vi "State_Waiting.vi"(8 "error in (no error)":errorcluster, 9 "Parameter":variant, 10 "Command":string, 11 "MB Slave Simulator Base in":refnum<class "MB Slave Simulator Base.lvclass">) -> (0 "error out":errorcluster, 2 "Debug Message":string, 3 "MB Slave Simulator Base out":refnum<class "MB Slave Simulator Base.lvclass">)   [LabVIEW 2021, in "MB Slave Simulator Base.lvclass"]
uses:
  MB Slave Simulator Base.lvclass
  C:/Program Files (x86)/National Instruments/LabVIEW 2021/user.lib/S2 Labs/Module Framework/Modules/Base/Module.lvclass
  C:/Program Files (x86)/National Instruments/LabVIEW 2021/user.lib/S2 Labs/Module Framework/Modules/Modbus/Modbus Slave Base/Modbus Slave Base.lvclass
  <userlib>/S2 Labs/CVT Toolkit/CVT.lvclass/CVT.ctl
  <userlib>/S2 Labs/Module Framework/Modules/Modbus/Modbus Slave Base/Modbus Slave Base.lvclass/Modbus Slave Base.ctl
  <userlib>/S2 Labs/Module Framework/Modules/Base/Module.lvclass/Module.ctl
  b9a700bc-881b-4d61-b18c-b62fca83ff33.vi
  d79701ff-d040-49f0-829a-e0d127d096ef.vi
  010a9ca9-5f64-4ce6-a378-2df25787252c.vi
  <userlib>/S2 Labs/Module Framework/Modules/Modbus/Modbus Slave Base/Read MB Ref.vi
  b9a700bc-881b-4d61-b18c-b62fca83ff33.vi/1553f4ce-967c-4f57-a913-5f155bf4374d.vi
  d79701ff-d040-49f0-829a-e0d127d096ef.vi/71b19a30-41bb-452f-8775-2cd3e07414b9.vi
  <userlib>/S2 Labs/Module Framework/Modules/Base/Read Module CVT.vi
  010a9ca9-5f64-4ce6-a378-2df25787252c.vi/71b19a30-41bb-452f-8775-2cd3e07414b9.vi
  <userlib>/S2 Labs/CVT Toolkit/Read CVT DVR.vi
  <userlib>/S2 Labs/CVT Toolkit/Variant Functions/Write Reserved Attributes.vi
  <userlib>/S2 Labs/CVT Toolkit/Variant Functions/Write Alias Attribute.vi
  <userlib>/S2 Labs/CVT Toolkit/Variant Functions/Write Unit Attribute.vi
  <userlib>/S2 Labs/CVT Toolkit/Variant Functions/Write Type Attribute.vi
  <userlib>/S2 Labs/CVT Toolkit/Variant Functions/Write Parms Attribute.vi
  <userlib>/S2 Labs/Module Framework/Modules/Base/Get Module CVT Ref.vi
  <userlib>/S2 Labs/Module Framework/Modules/Base/Trigger Logging Write.vi
  <userlib>/S2 Labs/Modbus Toolkit/Slave/S2L Modbus Slave.lvclass
  <userlib>/S2 Labs/CVT Toolkit/CVT.lvclass
  MB Slave Simulator Base.lvclass/MB Slave Simulator Base.ctl
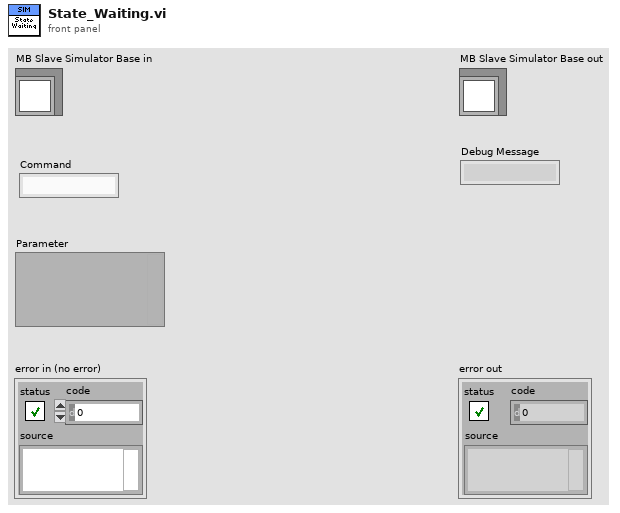
[diagram p1: front panel]
types:
  T1 = cluster{"daemon status":enum16{"Not Started", "Running", "Error", "Stopped"}, "daemon error":errorcluster, "connection count":u32, "connections":cluster{"Connected?":bool, "IP address":string, "connection error":errorcluster}[]}
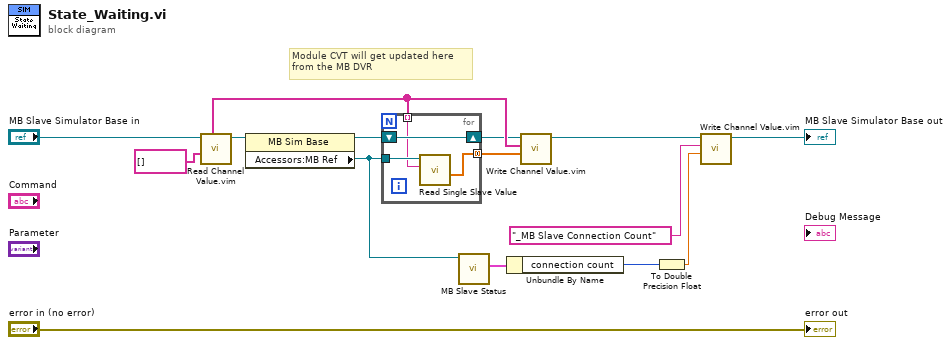
[diagram p0: block diagram]
diagram:
  # "Module CVT will get updated here\nfrom the MB DVR"
  n1 = call "Read Channel Value.vim"("Channel Label(s)"=string[] [], "Module in"="MB Slave Simulator Base in") -> ("Module out"=w9:refnum<class "MB Slave Simulator Base.lvclass">, "Channel Labels*"=w12:string[])  [unwired: 3 in, 5 out]
  n2 = property class="MB Sim Base"(reference=w9) -> (reference out=w10:refnum<class "MB Slave Simulator Base.lvclass">, "Accessors:MB Ref"=w15:refnum<class "S2L Modbus Slave.lvclass">)  [unwired: 1 in, 1 out]
  n3 = for {
    tunnel: w15 -> [w19]
    shift-right: [w18] -> w11
    shift-left: w10 -> [w18]
    tunnel: w12 -> [w17] mode=indexing
    tunnel: [w16] -> w13 mode=concatenating
    n4 = call-dynamic "Read Single Slave Value.vi"("Label"=w17, "S2L Modbus Slave in"=w19) -> ("Value (s)"=w16:dbl[])  [unwired: 4 in, 5 out]
  }
  n5 = call <userlib>:"MB Slave Status.vi"("S2L Modbus Slave in"=w15) -> ("MB Slave Status"=w4:T1)  [unwired: 8 in, 2 out]
  n6 = Unbundle By Name(w4) -> ("connection count"=w6:u32)
  n7 = call "Write Channel Value.vim"("value"=w13, "Channel Label(s)"=w12, "Module in"=w11) -> ("Module out"=w14:refnum<class "MB Slave Simulator Base.lvclass">)  [unwired: 6 in, 2 out]
  n8 = To Double Precision Float(number=w6) -> (double precision float=w7:dbl)
  n9 = call "Write Channel Value.vim"("value"=w7, "Channel Label(s)"="_MB Slave Connection Count", "Module in"=w14) -> ("Module out"=→"MB Slave Simulator Base out":refnum<class "MB Slave Simulator Base.lvclass">)  [unwired: 6 in, 2 out]
  "error out" <- "error in (no error)"
